vi "ACC Test.vi"() -> ()   [LabVIEW 2009]
panel:
  out "In Range?":bool
  in  "ACM SAMPLES":i32=1000
  in  "AMC RATE":dbl=1000.0
  out "ACELEROMETTER INPUTS":dynamicdata(graph)
  in  "U LIM X":dbl
  in  "L LIM X":dbl
  out "ACM X":dbl
  in  "stop":bool
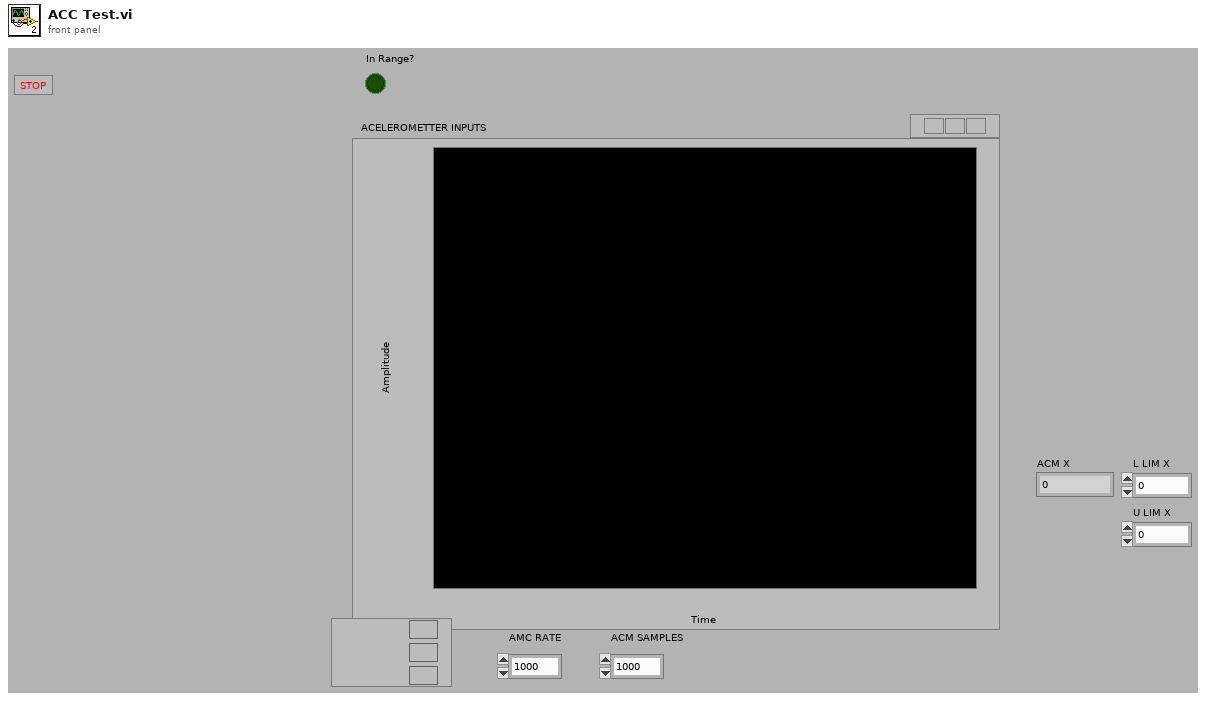
[diagram p1: front panel]
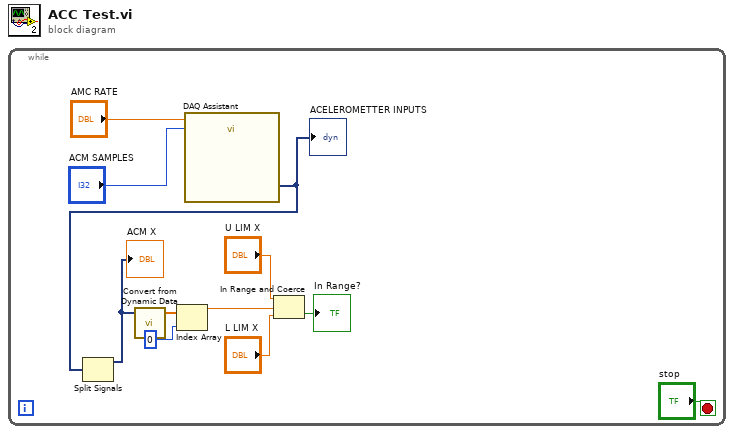
[diagram p0: block diagram]
diagram:
  n1 = while {
    stop <- "stop" stop-if-true
    n2 = call "DAQ Assistant"("rate"="AMC RATE", "number of samples"="ACM SAMPLES") -> ("data"=w4:dynamicdata)  [unwired: 15 in, 2 out]
    "ACELEROMETTER INPUTS" <- w4
    n3 = Split Signals(w4) -> (w7:dynamicdata)  [unwired: 3 in, 2 out]
    "ACM X" <- w7
    n4 = call "Convert from Dynamic Data"("Dynamic Data Type"=w7) -> ("Array"=w8:dbl[])  [unwired: 3 in]
    n5 = Index Array(array=w8, index=0) -> (element=w9:dbl)
    n6 = In Range and Coerce(upper limit="U LIM X", x=w9, lower limit="L LIM X") -> (In Range?=→"In Range?":bool)  [unwired: 1 out]
  }
